vi "Spectral Calculation (SubVI).vi"(0 "Measurement Cluster IN":T1, 1 "Write Spectral Data IN":bool, 6 "ON/OFF IN":bool) -> (20 "Measurement Cluster OUT":T1, 21 "Write Spectral Data OUT":bool, 22 "Calculated Data":dbl[](array[numeric]), 24 "Max Value":dbl format="%#_13g", 25 "Axis Title":string, 26 "ON/OFF OUT":bool)   [LabVIEW 2015]
uses:
  Measurement Cluster.ctl
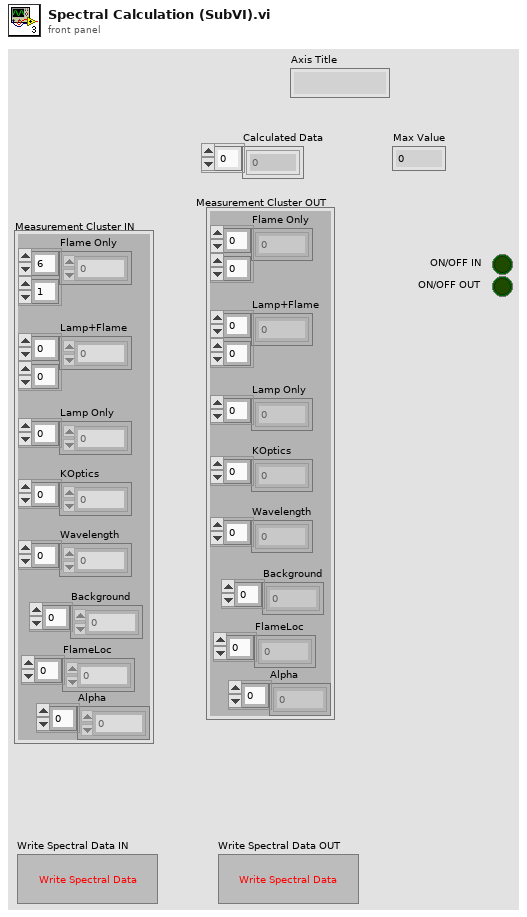
[diagram p1: front panel]
types:
  T1 = typedef "Measurement Cluster.ctl" = cluster{"Flame Only":dbl[][], "Lamp+Flame":dbl[][], "Lamp Only":dbl[], "KOptics":dbl[], "Wavelength":dbl[], "Background":dbl[], "FlameLoc":dbl[], "Alpha":dbl[]}
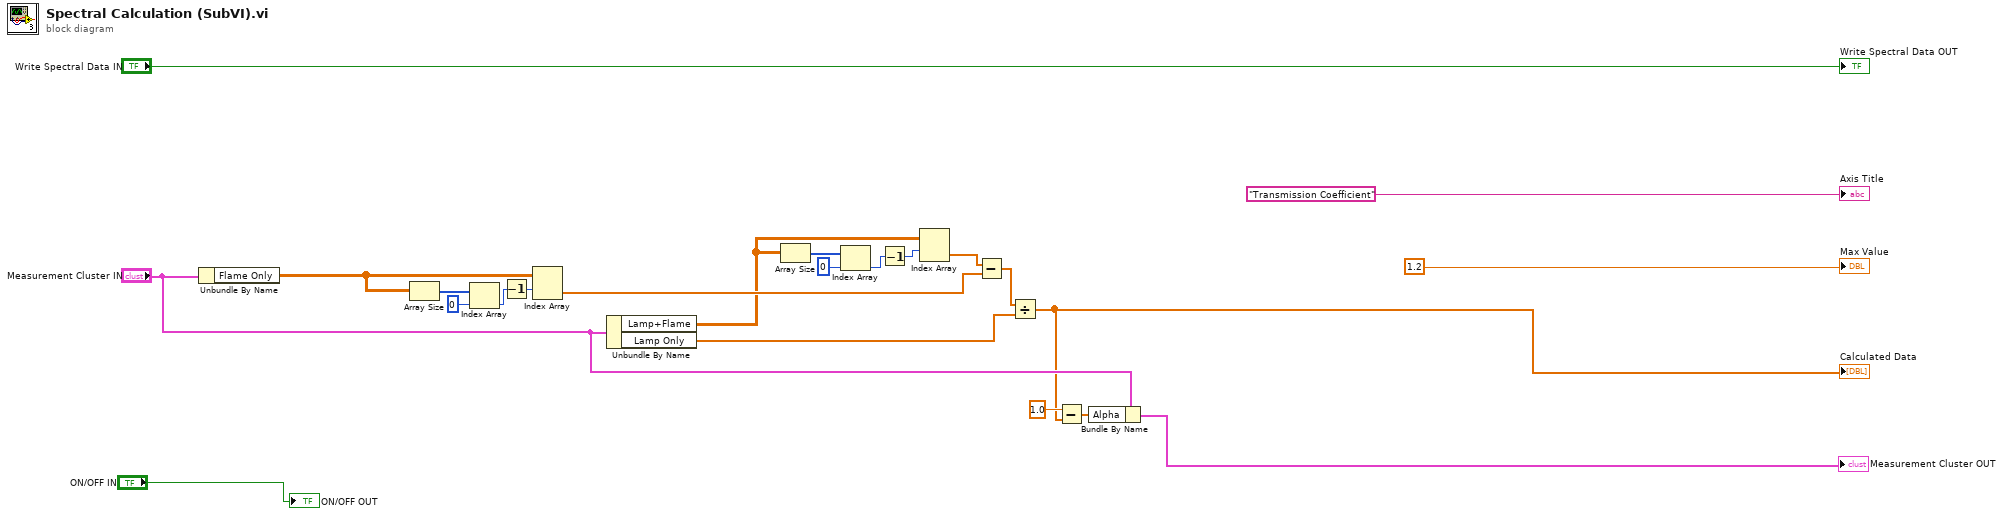
[diagram p0: block diagram]
diagram:
  n1 = Unbundle By Name("Measurement Cluster IN") -> ("Flame Only"=w13:dbl[][])
  n2 = Array Size(array=w13) -> (size(s)=w21:i32[])
  n3 = Index Array(array=w21, index=0) -> (element=w16:i32)
  n4 = Decrement(x=w16) -> (x-1=w17:i32)
  n5 = Index Array(array=w13, index (row)=w17) -> (element=w19:dbl[])  [unwired: 1 in]
  n6 = Unbundle By Name("Measurement Cluster IN") -> ("Lamp+Flame"=w7:dbl[][], "Lamp Only"=w4:dbl[])
  n7 = Array Size(array=w7) -> (size(s)=w10:i32[])
  n8 = Index Array(array=w10, index=0) -> (element=w8:i32)
  n9 = Decrement(x=w8) -> (x-1=w9:i32)
  n10 = Index Array(array=w7, index (row)=w9) -> (element=w6:dbl[])  [unwired: 1 in]
  n11 = Subtract(x=w6, y=w19) -> (x-y=w5:dbl[])
  n12 = Divide(x=w5, y=w4) -> (x/y=w2:dbl[])
  "Calculated Data" <- w2
  n13 = Subtract(x=1.0, y=w2) -> (x-y=w1:dbl[])
  n14 = Bundle By Name(cluster="Measurement Cluster IN", "Alpha"=w1) -> (→"Measurement Cluster OUT":T1)
  "Axis Title" <- "Transmission Coefficient"
  "Max Value" <- 1.2
  "Write Spectral Data OUT" <- "Write Spectral Data IN"
  "ON/OFF OUT" <- "ON/OFF IN"
